vi "optionsAcq_gainOpticalDetector.vi"(0 "reference":refnum<class "OSA200.lvclass">, 2 "gain_idx":u16=1, 4 "readWrite":enum16{"read", "write"}(ring), 5 "error in (no error)":errorcluster, 7 "ignore range violation (false)":bool) -> (14 "duplicate reference":refnum<class "OSA200.lvclass">, 15 "status":string, 16 "gain_idx  out":u16, 17 "gain_relative":dbl, 19 "error out":errorcluster)   [LabVIEW 2010, in "OSA200.lvclass"]
uses:
  OSA200.lvclass
  OSA.lvclass
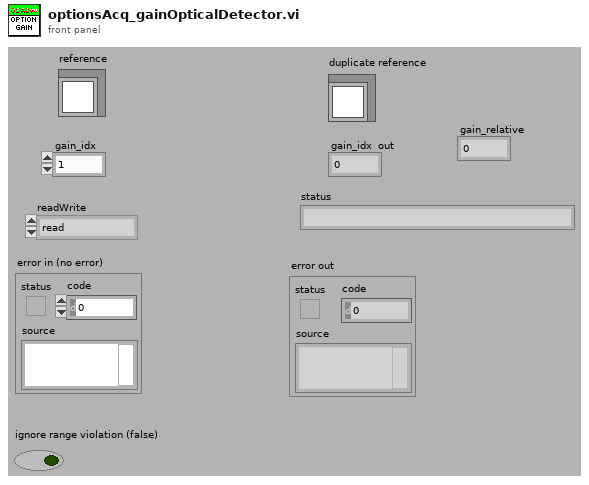
[diagram p1: front panel]
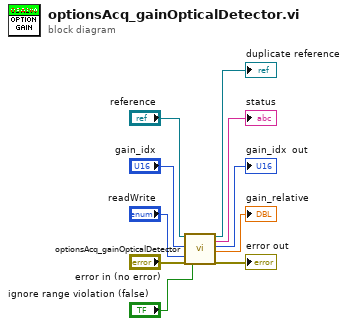
[diagram p0: block diagram]
diagram:
  n1 = call-parent "optionsAcq_gainOpticalDetector.vi"("reference"="reference", "gain_idx"="gain_idx", "readWrite"="readWrite", "error in (no error)"="error in (no error)", "ignore range violation (false)"="ignore range violation (false)") -> ("duplicate reference"=→"duplicate reference":refnum<class "OSA200.lvclass">, "status"=→"status":string, "gain_idx  out"=→"gain_idx  out":u16, "gain_relative"=→"gain_relative":dbl, "error out"=→"error out":errorcluster)  [unwired: 10 in]
